vi "test_serialize_deserialize.vi"   [LabVIEW 2020, in "NI_ADAS_Ethernet.lvlib"]
doc: "Version 0.1"
uses:
  NI_ADAS_Ethernet.lvlib
  Process Data.ctl
  Serialize Data.vi
  Deserialize Data.vi
  Serialize Data.vi/69b4f655-d322-486f-8d65-ee31f7d8c6ef.vi
  Deserialize Data.vi/5e2451cd-7b8c-4079-9add-41a600a01e16.vi
  <vilib>/ADAS Record/IODataPEF/Error/Error_CheckAndSetDllError.vi
  <vilib>/ADAS Record/IODataPEF/Error/Error_SetError.vi
  <vilib>/ADAS Record/IODataPEF/CfgMgr/GetPEFConfiguration_DefaultFlatFormat.vi
  <vilib>/ADAS Record/IODataPEF/Error/ErrorMgr.vi
  <vilib>/ADAS Record/CustomData/_Custom_RegisterType.vi
  <vilib>/addons/_JKI Toolkits/Caraya/classes/Test/Test.lvclass
  <vilib>/addons/_JKI Toolkits/Caraya/classes/Assert/Assert.lvclass
types:
  T1 = typedef "NI_ADAS_Ethernet.lvlib/Process Data.ctl" = cluster{"Timestamp":timestamp, "Bus Channel":u16, "Original Packet Length":u32, "Byte Array":u8[]}
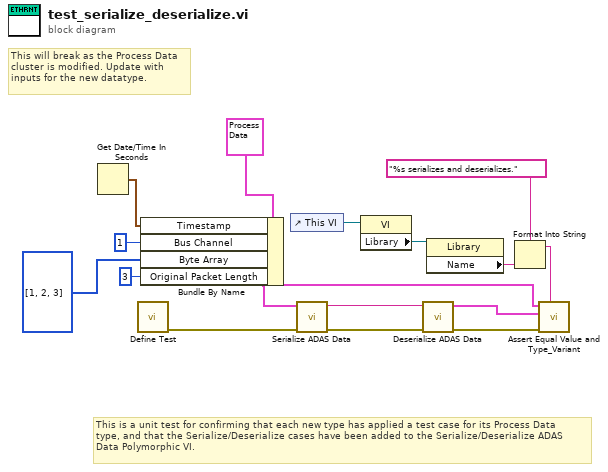
[diagram p0: block diagram]
diagram:
  # "This will break as the Process Data\ncluster is modified. Update with\ninputs for the new datatype."
  # "This is a unit test for confirming that each new type has applied a test case for its Process Data\ntype, and that the Serialize/Deserialize cases have been added to the Serialize/Deserialize ADAS\nData Polymorphic VI."
  n1 = Get Date/Time In Seconds() -> (seconds since 1Jan1904=w5:timestamp)
  n2 = call <vilib>:"Define Test.vi"() -> ("error out"=w11:errorcluster)  [unwired: 11 in]
  n3 = Bundle By Name(cluster=T1 {"Timestamp"=timestamp(0 s since 1904-01-01), "Bus Channel"=0, "Original Packet Length"=0, "Byte Array"=[]} ("Process Data in"), "Timestamp"=w5, "Bus Channel"=u16 1, "Byte Array"=u8[] [1, 2, 3], "Original Packet Length"=u32 3) -> (w2:T1)
  n4 = control-ref of="This VI"() -> (w16:refnum<vi>)
  n5 = call-poly "Serialize ADAS Data.vi"("error in (no error)"=w11, "Process Data"=w2) -> ("error out"=w10:errorcluster, "Flat Data out"=w9:string)  [unwired: 8 in]
  n6 = property class="VI"(reference=w16) -> ("Library"=w15:refnum<vi>)  [unwired: 1 in, 2 out]
  n7 = call-poly "Deserialize ADAS Data.vi"("error in (no error)"=w10, "Flat Data in"=w9) -> ("error out"=w7:errorcluster, "Process Data out"=w8:T1)  [unwired: 8 in]
  n8 = property class="Library"(reference=w15) -> ("Name"=w13:string)  [unwired: 1 in, 2 out]
  n9 = Format Into String(format string="%s serializes and deserializes.", w13) -> (resulting string=w12:string)  [unwired: 2 in, 1 out]
  n10 = call <vilib>:"Assert Equal Value and Type_Variant.vi"("Label"=w12, "error in (no error)"=w7, "Y"=w8, "X"=w2) -> ()  [unwired: 7 in, 1 out]
